vi "LDT Telescope Generate Target XML.vi"(8 "error in (no error)":errorcluster, 11 "Object out":T1) -> (0 "error out":errorcluster, 3 "XML String":string)   [LabVIEW 2022 SP3, in "LDT Telescope.lvclass"]
uses:
  LDT Telescope.lvclass
  typedefs/CC cluster Object.ctl
  typedefs/CC cluster sidereal rate.ctl
  typedefs/CC cluster RA and DEC.ctl
  typedefs/cc cluster muRA muDEC.ctl
  CC cluster Telescope Offsets.ctl
  Telescope cluster Equinox.ctl
  Telescope cluster Parallax.ctl
  Telescope cluster Rotator.ctl
  Telesope ring Frame.ctl
  Telescope.lvclass
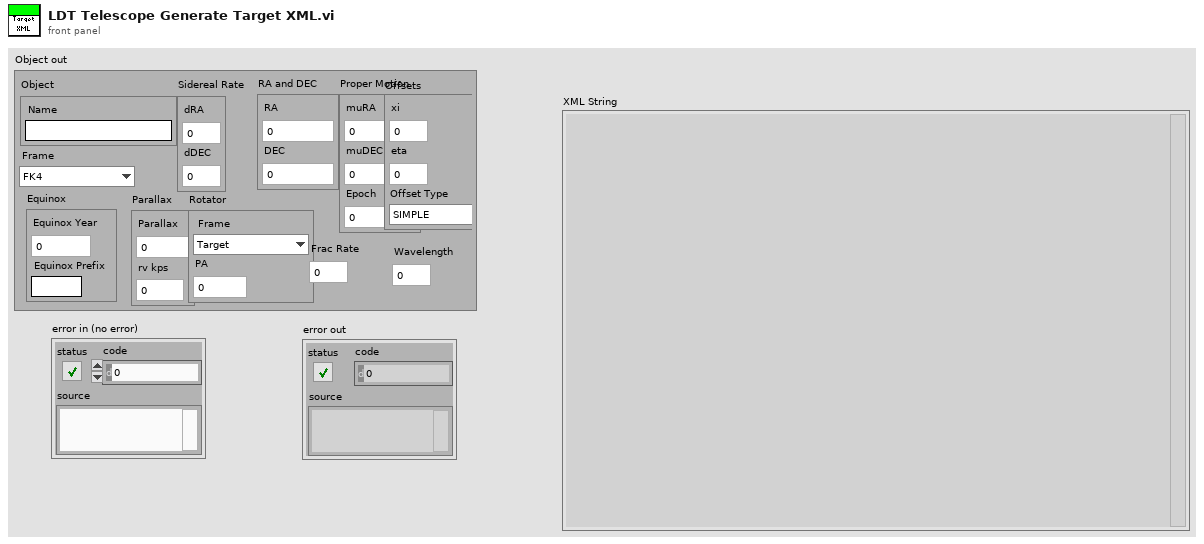
[diagram p1: front panel]
types:
  T1 = typedef "CC cluster Object.ctl" = cluster{"Object":cluster{"Name":string}, "Sidereal Rate":T2, "RA and DEC":T3, "Proper Motion":T4, "Offsets":T5, "Equinox":T6, "Parallax":T7, "Rotator":T8, "Frame":T9, "Frac Rate":dbl, "Wavelength":dbl}
  T2 = typedef "CC cluster sidereal rate.ctl" = cluster{"dRA":dbl, "dDEC":dbl}
  T3 = typedef "CC cluster RA and DEC.ctl" = cluster{"RA":dbl, "DEC":dbl}
  T4 = typedef "cc cluster muRA muDEC.ctl" = cluster{"muRA":dbl, "muDEC":dbl, "Epoch":dbl}
  T5 = typedef "CC cluster Telescope Offsets.ctl" = cluster{"xi":dbl, "eta":dbl, "Offset Type":enum16{"SIMPLE", "TPLANE", "PA"}}
  T6 = typedef "Telescope cluster Equinox.ctl" = cluster{"Equinox Year":i32, "Equinox Prefix":string}
  T7 = typedef "Telescope cluster Parallax.ctl" = cluster{"Parallax":dbl, "rv kps":dbl}
  T8 = typedef "Telescope cluster Rotator.ctl" = cluster{"Frame":enum16{"Target", "Fixed"}, "PA":dbl}
  T9 = typedef "Telesope ring Frame.ctl" = enum16{"FK4", "FK5", "APPT", "GAPPT", "AZEL"}
  T10 = cluster{"Degrees":dbl, "Arc Min":dbl, "Arc Sec":dbl}
  T11 = cluster{"hours":dbl, "Minutes":dbl, "seconds":dbl}
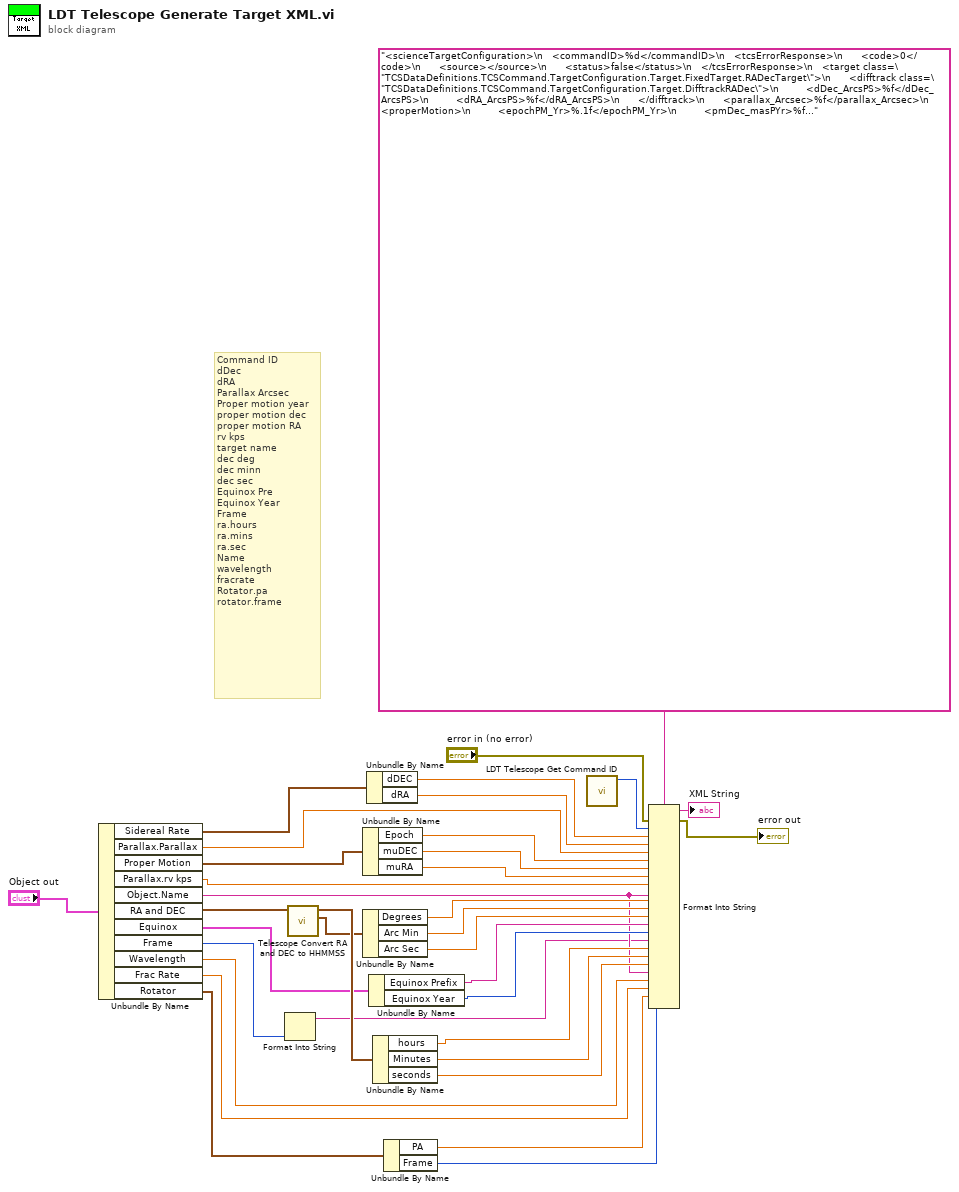
[diagram p0: block diagram]
diagram:
  # "Command ID\ndDec\ndRA\nParallax Arcsec\nProper motion year\nproper motion dec\nproper motion RA\nrv kps\ntarget name\ndec deg\ndec minn\ndec sec\nEquinox Pre\nEquinox Year\nFrame\nra.hours\nra.mins\nra.sec\nName\nwavelength\nfracrate\nRotator.pa\nrotator.frame"
  n1 = Unbundle By Name("Object out") -> ("Sidereal Rate"=w24:T2, "Parallax.Parallax"=w16:dbl, "Proper Motion"=w21:T4, "Parallax.rv kps"=w17:dbl, "Object.Name"=w8:string, "RA and DEC"=w32:T3, "Equinox"=w14:T6, "Frame"=w2:T9, "Wavelength"=w7:dbl, "Frac Rate"=w6:dbl, "Rotator"=w5:T8)
  n2 = Format Into String(w2) -> (resulting string=w1:string)  [unwired: 3 in, 1 out]
  n3 = call "Telescope Convert RA and DEC to HHMMSS.vi"("RA and DEC"=w32) -> ("Declination"=w31:T10, "Right Ascension"=w33:T11)  [unwired: 7 in, 2 out]
  n4 = Unbundle By Name(w21) -> ("Epoch"=w20:dbl, "muDEC"=w19:dbl, "muRA"=w18:dbl)
  n5 = Unbundle By Name(w31) -> ("Degrees"=w15:dbl, "Arc Min"=w30:dbl, "Arc Sec"=w29:dbl)
  n6 = Unbundle By Name(w24) -> ("dDEC"=w23:dbl, "dRA"=w22:dbl)
  n7 = Unbundle By Name(w14) -> ("Equinox Prefix"=w13:string, "Equinox Year"=w12:i32)
  n8 = Unbundle By Name(w33) -> ("hours"=w11:dbl, "Minutes"=w10:dbl, "seconds"=w9:dbl)
  n9 = Unbundle By Name(w5) -> ("PA"=w4:dbl, "Frame"=w3:enum16{"Target", "Fixed"})
  n10 = call "LDT Telescope Get Command ID.vi"() -> ("Command ID"=w27:i32)  [unwired: 10 in, 1 out]
  n11 = Format Into String(format string="<scienceTargetConfiguration>\n   <commandID>%d</commandID>\n   <tcsErrorResponse>\n      <code>0</code>\n      <source></source>\n      <status>false</status>\n   </tcsErrorResponse>\n   <target class=\"TCSDataDefinitions.TCSCommand.TargetConfiguration.Target.FixedTarget.RADecTarget\">\n      <difftrack class=\"TCSDataDefinitions.TCSCommand.TargetConfiguration.Target.DifftrackRADec\">\n         <dDec_ArcsPS>%f</dDec_ArcsPS>\n         <dRA_ArcsPS>%f</dRA_ArcsPS>\n      </difftrack>\n      <parallax_Arcsec>%f</parallax_Arcsec>\n      <properMotion>\n         <epochPM_Yr>%.1f</epochPM_Yr>\n         <pmDec_masPYr>%f</pmDec_masPYr>\n         <pmRA_masPYr>%f</pmRA_masPYr>\n      </properMotion>\n      <rv_kps>%f</rv_kps>\n      <targetName>%s</targetName>\n      <raDecParameters>\n         <declination>\n            <degreesDec>%f</degreesDec>\n            <minutesArc>%.1f</minutesArc>\n            <secondsArc>%.1f</secondsArc>\n         </declination>\n         <equinoxPrefix>%s</equinoxPrefix>\n         <equinoxYear>%.1f</equinoxYear>\n         <frame>%s</frame>\n         <ra>\n            <hours>%f</hours>\n            <minutesTime>%.1f</minutesTime>\n            <secondsTime>%.1f</secondsTime>\n         </ra>\n      </raDecParameters>\n   </target>\n   <targetConfigName>%s</targetConfigName>\n   <wl_microns>%f</wl_microns>\n   <fracrate>%f</fracrate>\n   <rotator>\n      <rotPA>%f</rotPA>\n      <rotatorFrame>%s</rotatorFrame>\n   </rotator>\n</scienceTargetConfiguration>", error in="error in (no error)", w27, w23, w22, w16, w20, w19, w18, w17, w8, w15, w30, w29, w13, w12, w1, w11, w10, w9, w8, w7, w6, w4, w3) -> (resulting string=→"XML String":string, error out=→"error out":errorcluster)  [unwired: 1 in]
